vi "Settings.vi"(5 "PSU Setup":T1={"Max Sweep(4.2K)"=0.003516666666666667, "Max Sweep(2.2K)"=0.003516666666666667, "Switch htr dly"=60.0, "O/P contactor?"=FALSE, "Max Field(4.2K)"=0.211, "Max Field(2.2K)"=0.211, "Description\n"="", "Settings.vi"=path "", "Max lead res"=0.5, "IO Info"={"Address"={"Com Port"=1, "ISOBUS Address"=1, "GPIB Address"=24, "Communication"=enum."ISOBUS"}, "Version"=enum."IPS"}, "Adjust shims"=FALSE} {"Max lead res" format="%.2f"; "Max Field(2.2K)" format="%.2f"; "Max Field(4.2K)" format="%.2f"; "Switch htr dly" format="%.2f"; "Max Sweep(2.2K)" format="%.2f"; "Max Sweep(4.2K)" format="%.2f"}) -> (0 "error out":errorcluster)   [LabVIEW 2016]
doc: "Opens the vi used to change the PS settimgs."
uses:
  Oxford Software/Oxsoft/PSAPPS.LLB/PSSetup.ctl
  Oxford Software/Oxsoft/PSSUBS.LLB/PSIO.ctl
  Oxford Software/Oxsoft/BUSGEN.LLB/OxfordAddress.ctl
panel:
  # "Press Shift F1 to edit this field"
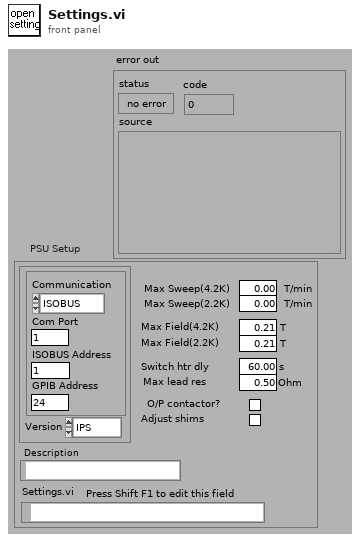
[diagram p1: front panel]
types:
  T1 = typedef "PSSetup.ctl" = cluster{"Max Sweep(4.2K)":dbl[unit], "Max Sweep(2.2K)":dbl[unit], "Switch htr dly":dbl[unit], "O/P contactor?":bool, "Max Field(4.2K)":dbl[unit], "Max Field(2.2K)":dbl[unit], "Description\n":string, "Settings.vi":path, "Max lead res":dbl[unit], "IO Info":T2, "Adjust shims":bool}
  T2 = typedef "PSIO.ctl" = cluster{"Address":T3, "Version":enum16{"PS", "IPS"}}
  T3 = typedef "OxfordAddress.ctl" = cluster{"Com Port":i32, "ISOBUS Address":i32, "GPIB Address":i16, "Communication":enum16{"RS232", "ISOBUS", "GPIB", "Gateway"}}
  T4 = cluster{string, "type string":i16[], "data string":string}
  T5 = cluster{string, "type string":i16[], "data string":string}[]
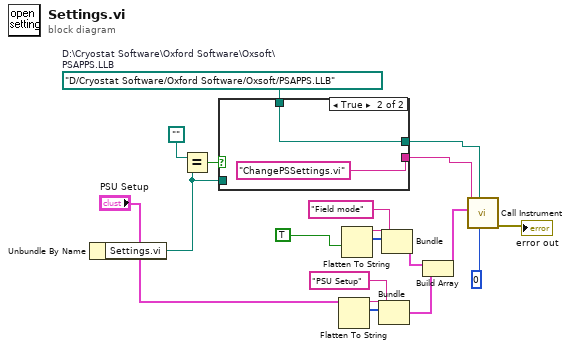
[diagram p0: block diagram]
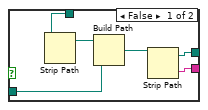
[diagram p2: hidden frame]
diagram:
  w1 = path "D:/Cryostat Software/Oxford Software/Oxsoft/PSAPPS.LLB"  # D:\Cryostat Software\Oxford Software\Oxsoft\PSAPPS.LLB
  n1 = Unbundle By Name("PSU Setup") -> ("Settings.vi"=w4:path)
  n2 = Equal?(x=path "", y=w4) -> (x = y?=w5:bool)
  n3 = case shown="True" w5 {
    tunnel: w4 -> [w21 _]
    tunnel: [w25 w26] -> w3
    tunnel: [w24 "ChangePSSettings.vi"] -> w2
    tunnel: w1 -> [w23 w26]
    frame False {
      n4 = Strip Path(path=w23) -> (stripped path=w22:path)  [unwired: 1 out]
      n5 = Build Path(base path=w22, name or relative path=w21) -> (appended path=w20:path)
      n6 = Strip Path(path=w20) -> (stripped path=w25:path, name=w24:string)
    }
    frame True {
    }
  }
  n7 = Flatten To String(anything="PSU Setup") -> (data string=w14:string, type string=w13:i16[])  [unwired: 3 in, 1 out]
  n8 = Flatten To String(anything=TRUE ("Field mode")) -> (data string=w19:string, type string=w18:i16[])  [unwired: 3 in, 1 out]
  n9 = Bundle("PSU Setup", "type string"=w13, "data string"=w14) -> (w10:T4)  [unwired: 1 in]
  n10 = Bundle("Field mode", "type string"=w18, "data string"=w19) -> (w11:T4)  [unwired: 1 in]
  n11 = Build Array(w11, w10) -> (w9:T5)
  n12 = call <vilib>:"Call Instrument.vi"("call mode (open,call,close:1)"=0, "VI path"=w3, "inputs"=w9, "VI name"=w2) -> ("error out"=→"error out":errorcluster)  [unwired: 6 in, 1 out]
